vi "Ctor.vi"(8 "error in (no error)":errorcluster) -> (0 "error out":errorcluster, 3 "Manager out":refnum<class "Manager.lvclass">)   [LabVIEW 2020, in "Stream-Simple-Msg.lvlib" / "Manager.lvclass"]
doc: "Initializes a new Messaging Manager instance. This must be called before using other members of the Manager class."
uses:
  Manager.lvclass
  Ref Data.ctl
  Callback.ctl
  Mapped Endpoint.ctl
  Endpoint/Endpoint.lvclass
  Format.ctl
  lv-stream/stream/Endpoint/Endpoint.lvclass
  State Callback.ctl
  Manager.lvclass/Manager.ctl
  Message/Message.lvclass
  Stream-Simple-Msg.lvlib
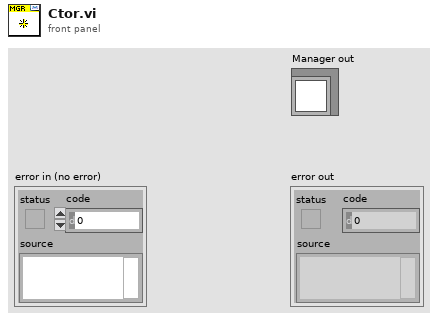
[diagram p1: front panel]
types:
  T1 = typedef "Stream-Simple-Msg.lvlib/Manager.lvclass/Ref Data.ctl" = cluster{"Message Callbacks":map{string, T2[]}, "Endpoints":map{string, T3}, "Stream Endpoints":refnum<class "Endpoint.lvclass">[], "State Callbacks":T5[], "Stream Formats":T4[]}
  T2 = typedef "Stream-Simple-Msg.lvlib/Manager.lvclass/Callback.ctl" = cluster{"VI":refnum<vi>, "Owner":refnum<class>}
  T3 = typedef "Stream-Simple-Msg.lvlib/Manager.lvclass/Mapped Endpoint.ctl" = cluster{"Msg Endpoint":refnum<class "Endpoint.lvclass">, "Format":T4}
  T4 = typedef "Stream-Simple-Msg.lvlib/Format.ctl" = enum16{"LabVIEW Binary", "JSON"}
  T5 = typedef "Stream-Simple-Msg.lvlib/Manager.lvclass/State Callback.ctl" = cluster{"Owner":refnum<class>, "VI":refnum<vi>, "Context":variant}
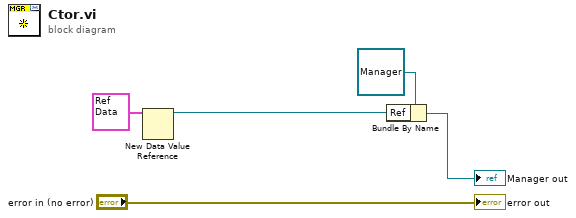
[diagram p0: block diagram]
diagram:
  n1 = New Data Value Reference(data value=T1 {"Message Callbacks"={}, "Endpoints"={}, "Stream Endpoints"=[], "State Callbacks"=[], "Stream Formats"=[]} ("Ref Data")) -> (data value reference=w1:refnum<data-value>)  [unwired: 1 in, 1 out]
  n2 = Bundle By Name(cluster=refnum<class "Manager.lvclass"> refnum ("Manager in"), "Ref"=w1) -> (→"Manager out":refnum<class "Manager.lvclass">)
  "error out" <- "error in (no error)"
